vi "Get Unique List of Test Channel Names.vi"(7 "UserName":string, 8 "error in (no error)":errorcluster, 10 "Other Constraints":T1[](array[typedef]), 11 "Test Name":string) -> (0 "error out":errorcluster, 3 "Unique List":string[](array[string]))   [LabVIEW 2011]
uses:
  eSearch Types.ctl
  DataFinder Comparisons.ctl
  Datafinder Query.ctl
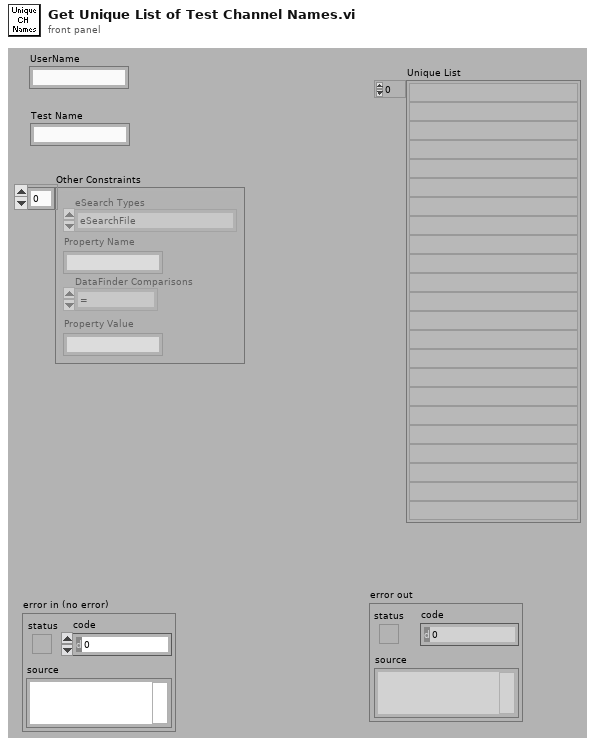
[diagram p1: front panel]
types:
  T1 = typedef "Datafinder Query.ctl" = cluster{"eSearch Types":T2, "Property Name":string, "DataFinder Comparisons":T3, "Property Value":string}
  T2 = typedef "eSearch Types.ctl" = enum16{"eSearchFile", "eSearchChannelGroup", "eSearchChannel"}
  T3 = typedef "DataFinder Comparisons.ctl" = enum16{"=", "<>", "<", "<=", ">", ">="}
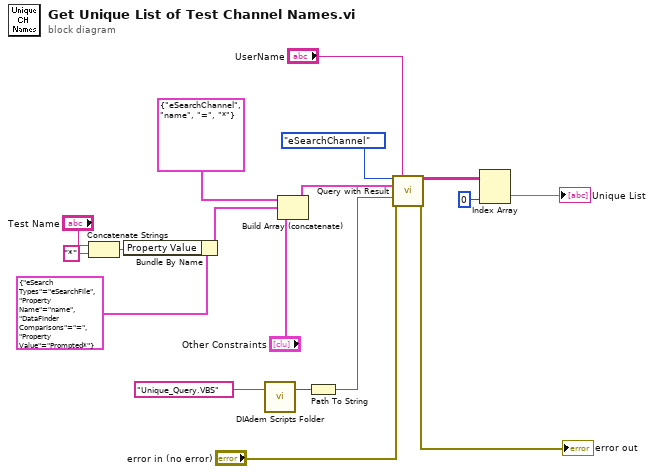
[diagram p0: block diagram]
diagram:
  n1 = Concatenate Strings("Test Name", "*" ("string")) -> (w8:string)
  n2 = Bundle By Name(cluster=T1 {"eSearch Types"=enum."eSearchFile", "Property Name"="name", "DataFinder Comparisons"=enum."=", "Property Value"="Prompted*"} ("Data Finder Parameters"), "Property Value"=w8) -> (w10:T1)
  n3 = call "DIAdem Scripts Folder.vi"("Relative Path (\"\" - Folder)"="Unique_Query.VBS" ("Query Name.vbs")) -> ("Scripts Folder"=w3:path)  [unwired: 2 out]
  n4 = Build Array (concatenate)(T1 {"eSearch Types"=enum."eSearchChannel", "Property Name"="name", "DataFinder Comparisons"=enum."=", "Property Value"="*"} ("Data Finder Parameters"), w10, "Other Constraints") -> (w13:T1[])
  n5 = Path To String(path=w3) -> (string=w2:string)
  n6 = call "Query with Result.vi"("eSearch Type"=eSearch_Types."eSearchChannel", "UserName"="UserName", "Search Parameters"=w13, "Query Name.vbs"=w2, "error in (no error)"="error in (no error)") -> ("Results"=w6:string[][], "error out"=→"error out":errorcluster)  [unwired: 9 out]
  n7 = Index Array(array=w6, index (col)=0 ("disabled index (col)")) -> (element=→"Unique List":string[])  [unwired: 1 in]
